vi "MoveToEndStop.vi"() -> ()   [LabVIEW 2021]
uses:
  <vilib>/MakerHub/LINX/Public/Peripherals/Digital/Digital Write 1 Chan.vi
  <vilib>/MakerHub/LINX/Public/Peripherals/Digital/Digital Write N Chans.vi
  <vilib>/MakerHub/LINX/Private/Local IO/LinxDigitalWrite.vi
  <vilib>/MakerHub/LINX/Public/Utilities/Check Channel.vi
  <vilib>/MakerHub/LINX/Public/Utilities/Open Serial.vi
  <vilib>/MakerHub/LINX/Private/Utilties/Generate Error.vi
  <vilib>/MakerHub/LINX/LMH-LINX.lvlib
panel:
  out "End Stop":bool
  in  "stop":bool
  in  "M1":bool
  in  "M0":bool
  out "error out":errorcluster
  in  "error in (no error)":errorcluster
  in  "Serial Port":refnum<visa-resource-name>="N/A"
  # "Function & M0 & M1\n ----------------------\nFull  Step:       0         0\n1/2   Step:       1         0\n1/8   Step:       0         1\n1/16 Step:       1         1"
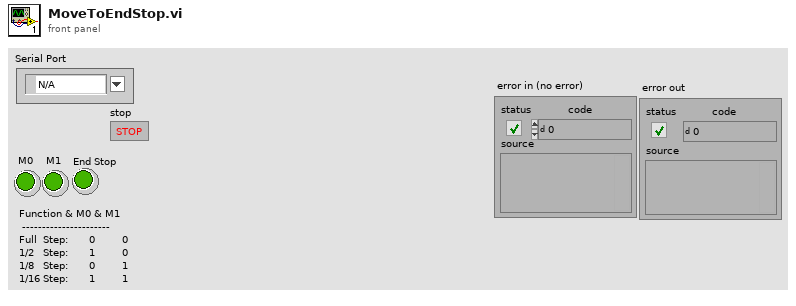
[diagram p1: front panel]
types:
  T1 = typedef "LMH-LINX.lvlib/LINX Ref.ctl" = cluster{"IO":T2, "Interface":T3, "LINX Device Config":T4}
  T2 = typedef "LMH-LINX.lvlib/Platform.ctl" = enum16{"Remote", "Local"}
  T3 = typedef "LMH-LINX.lvlib/Interface.ctl" = enum16{"Serial", "TCP"}
  T4 = typedef "LMH-LINX.lvlib/Device.lvlib/LINX Device Config.ctl" = cluster{"Interface":T3, "COM Port":refnum<visa-resource-name>, "TCP Configuration":T5, "Device Family":u8, "Device ID":u8, "Device Name":string, "TCP Ref":refnum<k5>, "Channels":T6}
  T5 = typedef "LMH-LINX.lvlib/Device.lvlib/TCP Config.ctl" = cluster{"IP Address":string, "Port":u16}
  T6 = typedef "LMH-LINX.lvlib/Channels.ctl" = cluster{"DI":u8[], "DO":u8[], "AI":u8[], "AO":u8[], "PWM":u8[], "QE":u8[], "UART":u8[], "I2C 2":u8[], "SPI":u8[], "CAN":u8[], "Servo":u8[], "AI Ref (V)":dbl, "AI Resolution (Bits)":u8, "AO Ref (V)":dbl, "AO Resolution (Bits)":u8}
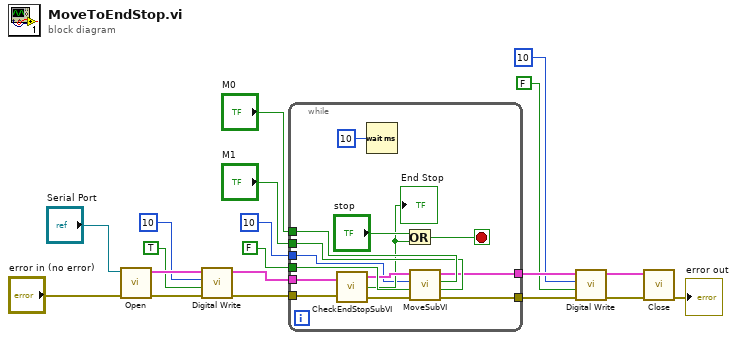
[diagram p0: block diagram]
diagram:
  n1 = call-poly <vilib>:"Open.vi"("Error In"="error in (no error)", "Serial Port"="Serial Port") -> ("Error Out"=w2:errorcluster, "LINX Resource"=w12:T1)  [unwired: 7 in, 1 out]
  n2 = call-poly <vilib>:"Digital Write.vi"("Error In"=w2, "Output Value"=TRUE, "DO Channel"=u8 10, "LINX Resource"=w12) -> ("Error Out"=w1:errorcluster, "LINX Resource"=w11:T1)  [unwired: 6 in]
  n3 = while {
    tunnel: FALSE ("Direction") -> [w33]
    tunnel: "M0" -> [w32]
    tunnel: "M1" -> [w31]
    tunnel: [w29] -> w10
    tunnel: [w27] -> w8
    tunnel: u32 10 ("Number of Steps") -> [w23]
    tunnel: w11 -> [w21]
    tunnel: w1 -> [w20]
    stop <- w25 stop-if-true
    n4 = call "CheckEndStopSubVI.vi"("LINX Resource"=w21, "error in (no error)"=w20) -> ("LINX Resource 2"=w30:T1, "DI Value"=w24:bool, "error out"=w28:errorcluster)
    "End Stop" <- w24
    n5 = Wait (ms)(milliseconds to wait=u32 10) -> ()  [unwired: 1 out]
    n6 = Or(x="stop", y=w24) -> (x .or. y?=w25:bool)
    n7 = call "MoveSubVI.vi"("M1"=w31, "M0"=w32, "error in (no error)"=w28, "Direction"=w33, "Number of Steps"=w23, "LINX Resource"=w30) -> ("error out"=w27:errorcluster, "LINX Resource 2"=w29:T1)
  }
  n8 = call-poly <vilib>:"Digital Write.vi"("Error In"=w8, "Output Value"=FALSE, "DO Channel"=u8 10, "LINX Resource"=w10) -> ("Error Out"=w7:errorcluster, "LINX Resource"=w9:T1)  [unwired: 6 in]
  n9 = call <vilib>:"Close.vi"("Error In"=w7, "LINX Resource"=w9) -> ("Error Out"=→"error out":errorcluster)  [unwired: 9 in]
